vi "SERVER GERAL.vi"() -> ()   [LabVIEW 2019]
uses:
  Strict_Type_Def_Valores_Instrumentos.ctl
panel:
  in  "NOMES":string[](array[string])
  in  "Valores_Instrumentos":T1 {"JG_AR" format="%#_6e"; "DeltaP_K" format="%#_6e"; "DeltaP_W" format="%#_6e"; "Diâmetro Tubulação [m]" format="%#_6e"; "PC-TQ-TD" format="%#_6e"; "PC-TQ-TI" format="%#_6e"; "PC-TQ-GP" format="%#_6e"; "PC-TQ-PV" format="%#_6e"; "PC-TQ-SP" format="%#_6e"; "PC-TQ-OV" format="%#_6e"; "SPW-WR-VEL" format="%#_6e"; "SPK-WR-VEL" format="%#_6e"; "SKM-PC-TQ" format="%#_6e"; "SKM-FC-KF" format="%#_6e"; "SKM-FC-WF" format="%#_6e"; "SKM-FC-AR" format="%#_6e"; "SKM-TI-KF_COR" format="%#_6e"; "SKS-LC-K" format="%#_6e"; "SPK-RD-CRT" format="%#_6e"; "SPW-RD-CRT" format="%#_6e"; "SKM-FIC-AR_COR" format="%#_6e"; "SKM-FIC-KF_COR" format="%#_6e"; "SKM-AI-AR_COR" format="%#_6e"; "SKM-AI-KF_COR" format="%#_6e"; "SKM-TI-AR_COR" format="%#_6e"; "SKM-TI-KF" format="%#_6e"; "SPW-RD-VEL" format="%#_6e"; "SPK-RD-VEL" format="%#_6e"; "SKS-LC-W" format="%#_6e"; "SIT-PI-002" format="%#_6e"; "SKM-FI-WF" format="%#_6e"; "SKM-TI-WF" format="%#_6e"; "SKM-PI-BAR" format="%#_6e"; "SKM-PI-LAM" format="%#_6e"; "SMA-PI-LAM" format="%#_6e"; "SMA-TI-LAM" format="%#_6e"; "SKM-PI-TQ" format="%#_6e"; "SKM-TI-TQ" format="%#_6e"}
  in  "stop":bool
  # "SKID MEDI敲O - LEITURA"
  # "SKID MEDI敲O - ESCRITA"
  # "SKID BOMBA - ESCRITA"
  # "SKID BOMBA - LEITURA"
  # "SKID SEPARA敲O - LEITURA"
  # "SKID INJE敲O - LEITURA"
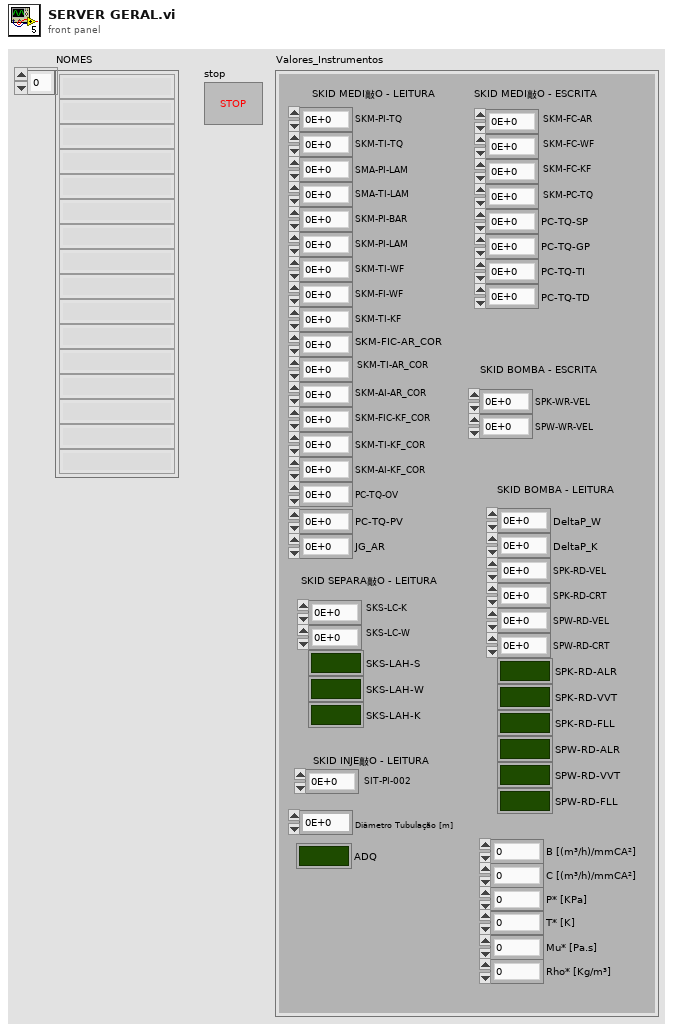
[diagram p1: front panel]
types:
  T1 = typedef "Strict_Type_Def_Valores_Instrumentos.ctl" = cluster{"SKM-TI-TQ":dbl, "SKM-PI-TQ":dbl, "SMA-TI-LAM":dbl, "SMA-PI-LAM":dbl, "SKM-PI-LAM":dbl, "SKM-PI-BAR":dbl, "SKM-TI-WF":dbl, "SKM-FI-WF":dbl, "SIT-PI-002":dbl, "SKS-LC-W":dbl, "SPK-RD-VEL":dbl, "SPW-RD-VEL":dbl, "SKM-TI-KF":dbl, "SKM-TI-AR_COR":dbl, "SKM-AI-KF_COR":dbl, "SKM-AI-AR_COR":dbl, "SKM-FIC-KF_COR":dbl, "SKM-FIC-AR_COR":dbl, "SPW-RD-CRT":dbl, "SPK-RD-CRT":dbl, "SKS-LC-K":dbl, "SKM-TI-KF_COR":dbl, "SKM-FC-AR":dbl, "SKM-FC-WF":dbl, "SKM-FC-KF":dbl, "SKM-PC-TQ":dbl, "SPK-WR-VEL":dbl, "SPW-WR-VEL":dbl, "SPK-RD-ALR":bool, "SPK-RD-VVT":bool, "SPK-RD-FLL":bool, "SPW-RD-ALR":bool, "SPW-RD-VVT":bool, "SPW-RD-FLL":bool, "PC-TQ-OV":dbl, "PC-TQ-SP":dbl, "PC-TQ-PV":dbl, "PC-TQ-GP":dbl, "PC-TQ-TI":dbl, "PC-TQ-TD":dbl, "SKS-LAH-S":bool, "SKS-LAH-W":bool, "SKS-LAH-K":bool, "Diâmetro Tubulação [m]":dbl, "DeltaP_W":dbl, "DeltaP_K":dbl, "ADQ":bool, "JG_AR":dbl, "B [(m³/h)/mmCA²]":dbl, "C [(m³/h)/mmCA²]":dbl, "P* [KPa]":dbl, "T* [K]":dbl, "Mu* [Pa.s] ":dbl, "Rho* [Kg/m³]":dbl}
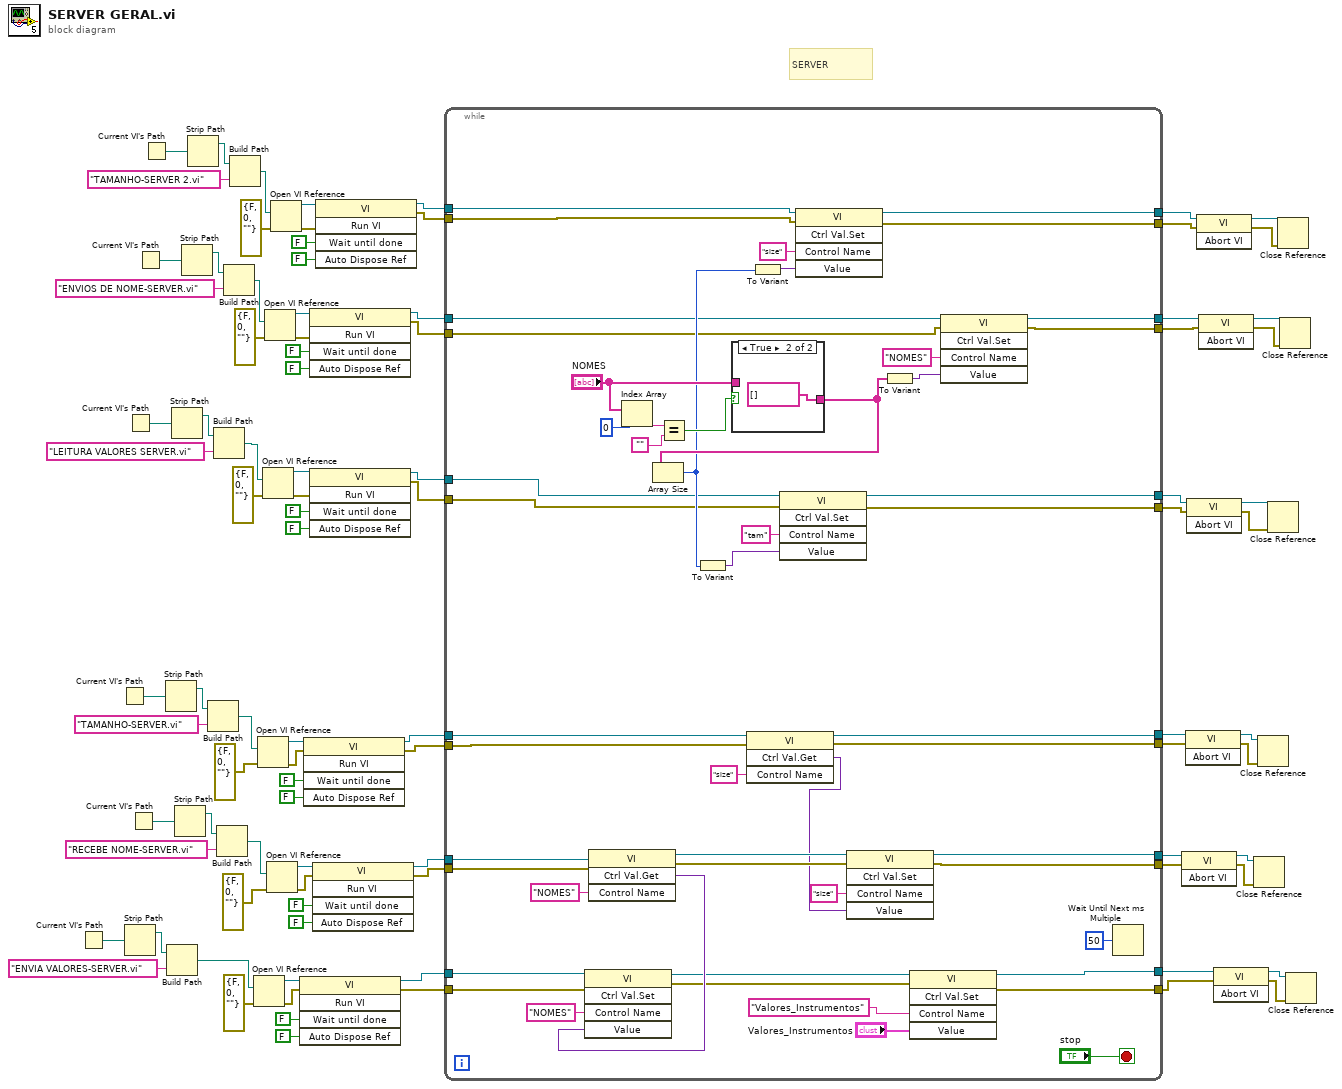
[diagram p0: block diagram]
diagram:
  # "SERVER"
  n1 = Current VI's Path() -> (path=w64:path)
  n2 = Current VI's Path() -> (path=w56:path)
  n3 = Strip Path(path=w64) -> (stripped path=w63:path)  [unwired: 1 out]
  n4 = Current VI's Path() -> (path=w32:path)
  n5 = Current VI's Path() -> (path=w68:path)
  n6 = Current VI's Path() -> (path=w29:path)
  n7 = Current VI's Path() -> (path=w37:path)
  n8 = Strip Path(path=w56) -> (stripped path=w55:path)  [unwired: 1 out]
  n9 = Build Path(base path=w63, name or relative path="ENVIA VALORES-SERVER.vi") -> (appended path=w61:path)
  n10 = Strip Path(path=w32) -> (stripped path=w33:path)  [unwired: 1 out]
  n11 = Strip Path(path=w68) -> (stripped path=w67:path)  [unwired: 1 out]
  n12 = Strip Path(path=w29) -> (stripped path=w30:path)  [unwired: 1 out]
  n13 = Strip Path(path=w37) -> (stripped path=w38:path)  [unwired: 1 out]
  n14 = Build Path(base path=w55, name or relative path="TAMANHO-SERVER.vi") -> (appended path=w53:path)
  n15 = Build Path(base path=w33, name or relative path="LEITURA VALORES SERVER.vi") -> (appended path=w34:path)
  n16 = Build Path(base path=w67, name or relative path="RECEBE NOME-SERVER.vi") -> (appended path=w65:path)
  n17 = Build Path(base path=w30, name or relative path="ENVIOS DE NOME-SERVER.vi") -> (appended path=w31:path)
  n18 = Build Path(base path=w38, name or relative path="TAMANHO-SERVER 2.vi") -> (appended path=w39:path)
  n19 = Open VI Reference(vi path=w61, error in (no error)=errorcluster {"status"=FALSE, "code"=0, "source"=""}) -> (vi reference=w83:refnum<vi>, error out=w82:errorcluster)  [unwired: 4 in]
  n20 = Open VI Reference(vi path=w53, error in (no error)=errorcluster {"status"=FALSE, "code"=0, "source"=""}) -> (vi reference=w60:refnum<vi>, error out=w59:errorcluster)  [unwired: 4 in]
  n21 = Open VI Reference(vi path=w34, error in (no error)=errorcluster {"status"=FALSE, "code"=0, "source"=""}) -> (vi reference=w28:refnum<vi>, error out=w27:errorcluster)  [unwired: 4 in]
  n22 = Open VI Reference(vi path=w31, error in (no error)=errorcluster {"status"=FALSE, "code"=0, "source"=""}) -> (vi reference=w25:refnum<vi>, error out=w26:errorcluster)  [unwired: 4 in]
  n23 = Open VI Reference(vi path=w65, error in (no error)=errorcluster {"status"=FALSE, "code"=0, "source"=""}) -> (vi reference=w90:refnum<vi>, error out=w89:errorcluster)  [unwired: 4 in]
  n24 = Open VI Reference(vi path=w39, error in (no error)=errorcluster {"status"=FALSE, "code"=0, "source"=""}) -> (vi reference=w35:refnum<vi>, error out=w36:errorcluster)  [unwired: 4 in]
  n25 = invoke class="VI" method="Run VI"(reference=w83, error in=w82, "Wait until done"=FALSE ("Wait Until Done"), "Auto Dispose Ref"=FALSE ("Auto Dispose Reference")) -> (reference out=w78:refnum<vi>, error out=w77:errorcluster)  [unwired: 1 in, 3 out]
  n26 = invoke class="VI" method="Run VI"(reference=w60, error in=w59, "Wait until done"=FALSE ("Wait Until Done"), "Auto Dispose Ref"=FALSE ("Auto Dispose Reference")) -> (reference out=w49:refnum<vi>, error out=w47:errorcluster)  [unwired: 1 in, 3 out]
  n27 = invoke class="VI" method="Run VI"(reference=w25, error in=w26, "Wait until done"=FALSE ("Wait Until Done"), "Auto Dispose Ref"=FALSE ("Auto Dispose Reference")) -> (reference out=w4:refnum<vi>, error out=w3:errorcluster)  [unwired: 1 in, 3 out]
  n28 = invoke class="VI" method="Run VI"(reference=w28, error in=w27, "Wait until done"=FALSE ("Wait Until Done"), "Auto Dispose Ref"=FALSE ("Auto Dispose Reference")) -> (reference out=w2:refnum<vi>, error out=w1:errorcluster)  [unwired: 1 in, 3 out]
  n29 = invoke class="VI" method="Run VI"(reference=w90, error in=w89, "Wait until done"=FALSE ("Wait Until Done"), "Auto Dispose Ref"=FALSE ("Auto Dispose Reference")) -> (reference out=w85:refnum<vi>, error out=w84:errorcluster)  [unwired: 1 in, 3 out]
  n30 = invoke class="VI" method="Run VI"(reference=w35, error in=w36, "Wait until done"=FALSE ("Wait Until Done"), "Auto Dispose Ref"=FALSE ("Auto Dispose Reference")) -> (reference out=w6:refnum<vi>, error out=w5:errorcluster)  [unwired: 1 in, 3 out]
  n31 = while {
    tunnel: [w124] -> w70
    tunnel: w85 -> [w137]
    tunnel: w84 -> [w136]
    tunnel: [w123] -> w69
    tunnel: w78 -> [w140]
    tunnel: w77 -> [w139]
    tunnel: [w131] -> w76
    tunnel: [w130] -> w75
    tunnel: [w119] -> w50
    tunnel: w49 -> [w121]
    tunnel: [w118] -> w48
    tunnel: w47 -> [w120]
    tunnel: [w102] -> w12
    tunnel: [w101] -> w11
    tunnel: [w100] -> w10
    tunnel: [w99] -> w9
    tunnel: [w98] -> w8
    tunnel: [w97] -> w7
    tunnel: w6 -> [w96]
    tunnel: w5 -> [w95]
    tunnel: w4 -> [w94]
    tunnel: w3 -> [w93]
    tunnel: w2 -> [w92]
    tunnel: w1 -> [w91]
    stop <- "stop" stop-if-true
    n32 = invoke class="VI" method="Ctrl Val.Get"(reference=w137, error in=w136, "Control Name"="NOMES") -> (reference out=w126:refnum<vi>, error out=w125:errorcluster, "Get Control Value Variant"=w134:variant)  [unwired: 1 in, 1 out]
    n33 = invoke class="VI" method="Ctrl Val.Set"(reference=w140, error in=w139, "Control Name"="NOMES", "Value"=w134) -> (reference out=w133:refnum<vi>, error out=w132:errorcluster)  [unwired: 1 in, 3 out]
    n34 = Index Array(array="NOMES", index=0) -> (element=w108:string)
    n35 = Equal?(x=w108, y="") -> (x = y?=w106:bool)
    n36 = case shown="True" w106 {
      tunnel: [w142 string[] [] ("NOMES")] -> w110
      tunnel: "NOMES" -> [w142 _]
      frame False {
      }
      frame True {
      }
    }
    n37 = Array Size(array=w110) -> (size(s)=w103:i32)
    n38 = To Variant(anything=w103) -> (Variant=w114:variant)
    n39 = invoke class="VI" method="Ctrl Val.Get"(reference=w121, error in=w120, "Control Name"="size") -> (reference out=w119:refnum<vi>, error out=w118:errorcluster, "Get Control Value Variant"=w116:variant)  [unwired: 1 in, 1 out]
    n40 = To Variant(anything=w103) -> (Variant=w104:variant)
    n41 = invoke class="VI" method="Ctrl Val.Set"(reference=w92, error in=w91, "Control Name"="tam", "Value"=w114) -> (reference out=w98:refnum<vi>, error out=w97:errorcluster)  [unwired: 1 in, 3 out]
    n42 = invoke class="VI" method="Ctrl Val.Set"(reference=w96, error in=w95, "Control Name"="size", "Value"=w104) -> (reference out=w102:refnum<vi>, error out=w101:errorcluster)  [unwired: 1 in, 3 out]
    n43 = invoke class="VI" method="Ctrl Val.Set"(reference=w126, error in=w125, "Control Name"="size", "Value"=w116) -> (reference out=w124:refnum<vi>, error out=w123:errorcluster)  [unwired: 1 in, 3 out]
    n44 = To Variant(anything=w110) -> (Variant=w112:variant)
    n45 = invoke class="VI" method="Ctrl Val.Set"(reference=w133, error in=w132, "Control Name"="Valores_Instrumentos", "Value"="Valores_Instrumentos") -> (reference out=w131:refnum<vi>, error out=w130:errorcluster)  [unwired: 1 in, 3 out]
    n46 = invoke class="VI" method="Ctrl Val.Set"(reference=w94, error in=w93, "Control Name"="NOMES", "Value"=w112) -> (reference out=w100:refnum<vi>, error out=w99:errorcluster)  [unwired: 1 in, 3 out]
    n47 = Wait Until Next ms Multiple(millisecond multiple=u32 50) -> ()  [unwired: 1 out]
  }
  n48 = invoke class="VI" method="Abort VI"(reference=w70, error in=w69) -> (reference out=w72:refnum<vi>, error out=w71:errorcluster)  [unwired: 1 in, 1 out]
  n49 = invoke class="VI" method="Abort VI"(reference=w50, error in=w48) -> (reference out=w52:refnum<vi>, error out=w51:errorcluster)  [unwired: 1 in, 1 out]
  n50 = invoke class="VI" method="Abort VI"(reference=w8, error in=w7) -> (reference out=w41:refnum<vi>, error out=w42:errorcluster)  [unwired: 1 in, 1 out]
  n51 = invoke class="VI" method="Abort VI"(reference=w12, error in=w11) -> (reference out=w44:refnum<vi>, error out=w45:errorcluster)  [unwired: 1 in, 1 out]
  n52 = invoke class="VI" method="Abort VI"(reference=w10, error in=w9) -> (reference out=w40:refnum<vi>, error out=w43:errorcluster)  [unwired: 1 in, 1 out]
  n53 = invoke class="VI" method="Abort VI"(reference=w76, error in=w75) -> (reference out=w74:refnum<vi>, error out=w73:errorcluster)  [unwired: 1 in, 1 out]
  n54 = Close Reference(reference=w72, error in (no error)=w71) -> ()  [unwired: 1 out]
  n55 = Close Reference(reference=w52, error in (no error)=w51) -> ()  [unwired: 1 out]
  n56 = Close Reference(reference=w41, error in (no error)=w42) -> ()  [unwired: 1 out]
  n57 = Close Reference(reference=w44, error in (no error)=w45) -> ()  [unwired: 1 out]
  n58 = Close Reference(reference=w40, error in (no error)=w43) -> ()  [unwired: 1 out]
  n59 = Close Reference(reference=w74, error in (no error)=w73) -> ()  [unwired: 1 out]
